vi "SRV_Update Streaming States VIG.vi"(7 "Enabled":bool, 9 "Data":string, 12 "Streaming Modes":T1) -> ()   [LabVIEW 2009]
uses:
  SRV_Streaming Modes.ctl
  SRV_Streaming State.ctl
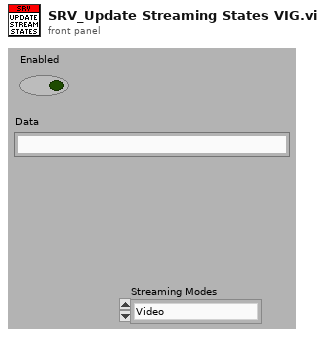
[diagram p1: front panel]
types:
  T1 = typedef "SRV_Streaming Modes.ctl" = enum16{"Video", "Sensors"}
  T2 = typedef "SRV_Streaming State.ctl" = cluster{"Enabled":bool, "Data":string}
  T3 = typedef "SRV_Streaming States.ctl" = cluster{"Video":T2, "Sensors":T2}
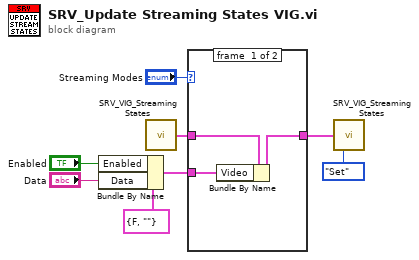
[diagram p0: block diagram]
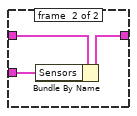
[diagram p2: hidden frame]
diagram:
  n1 = Bundle By Name(cluster=T2 {"Enabled"=FALSE, "Data"=""} ("Streaming State"), "Enabled"="Enabled", "Data"="Data") -> (w3:T2)
  n2 = call "SRV_VIG_Streaming States.vi"() -> ("Streaming States out"=w7:T3)  [unwired: 15 in]
  n3 = case shown="\"Video\"" "Streaming Modes" {
    tunnel: w7 -> [w11 w14]
    tunnel: [w10 w13] -> w6
    tunnel: w3 -> [w9 w12]
    frame #0 {
      n4 = Bundle By Name(cluster=w11, "Video"=w9) -> (w10:T3)
    }
    frame #1 {
      n5 = Bundle By Name(cluster=w14, "Sensors"=w12) -> (w13:T3)
    }
  }
  n6 = call "SRV_VIG_Streaming States.vi"("Streaming States"=w6, "Method (Get)"=enum16{"Get", "Set"}."Set") -> ()  [unwired: 13 in, 1 out]
